vi "Build Metadata String.vi"(11 "Macro Config":T1) -> (3 "Metadata":string)   [LabVIEW 2020, in "MacroAssert.lvlib"]
doc: "Builds a metadata string from <B>Macro Config</B> to be displayed to the user."
uses:
  MacroAssert.lvlib
  CTLs/Macro Config V3.ctl
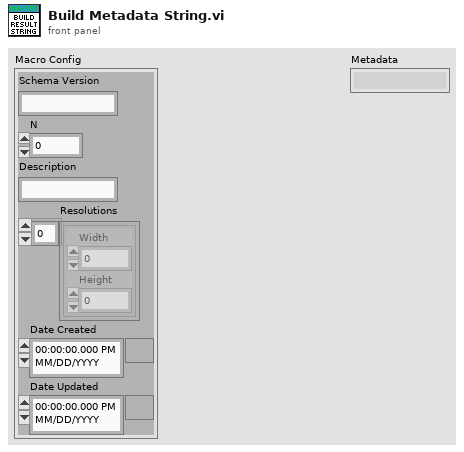
[diagram p1: front panel]
types:
  T1 = typedef "MacroAssert.lvlib/Macro Config V3.ctl" = cluster{"Schema Version":string, "N":i32, "Description":string, "Resolutions":cluster{"Width":i16, "Height":i16}[], "Date Created":timestamp, "Date Updated":timestamp}
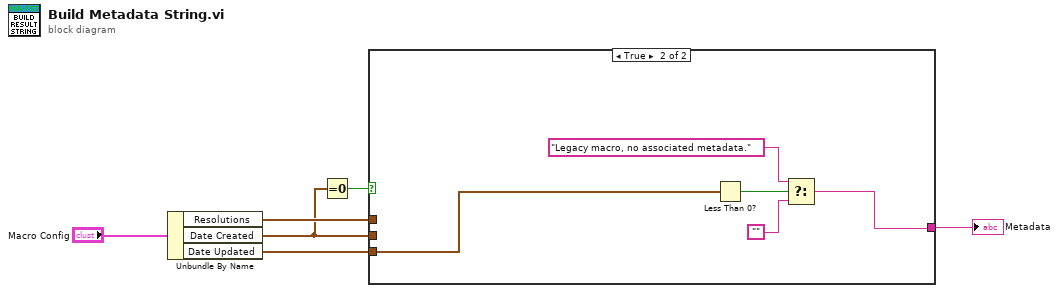
[diagram p0: block diagram]
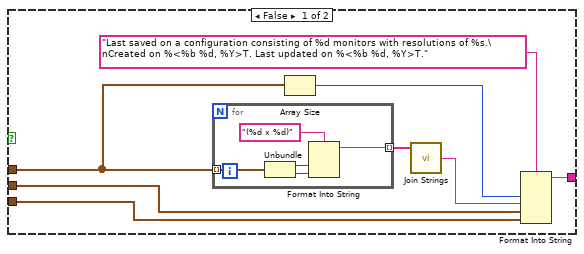
[diagram p2: hidden frame]
diagram:
  n1 = Unbundle By Name("Macro Config") -> ("Resolutions"=w5:cluster{"Width":i16, "Height":i16}[], "Date Created"=w2:timestamp, "Date Updated"=w6:timestamp)
  n2 = Equal To 0?(x=w2) -> (x = 0?=w3:bool)
  n3 = case shown="True" w3 {
    tunnel: w6 -> [w13 w24]
    tunnel: w2 -> [w12 _]
    tunnel: w5 -> [w10 _]
    tunnel: [w7 w20] -> w4
    frame False {
      n4 = for {
        tunnel: w10 -> [w18] mode=indexing
        tunnel: [w15] -> w9 mode=indexing
        n5 = Unbundle(w18) -> ("Width"=w16:i16, "Height"=w17:i16)
        n6 = Format Into String(format string="(%d x %d)", w16, w17) -> (resulting string=w15:string)  [unwired: 2 in, 1 out]
      }
      n7 = Array Size(array=w10) -> (size(s)=w11:i32)
      n8 = call <vilib>:"Join Strings.vi"("Strings In"=w9) -> ("String"=w8:string)  [unwired: 2 in]
      n9 = Format Into String(format string="Last saved on a configuration consisting of %d monitors with resolutions of %s.\nCreated on %<%b %d, %Y>T. Last updated on %<%b %d, %Y>T.", w11, w8, w12, w13) -> (resulting string=w7:string)  [unwired: 2 in, 1 out]
    }
    frame True {
      n10 = Less Than 0?(x=w24) -> (x < 0?=w23:bool)
      n11 = Select(t="Legacy macro, no associated metadata.", s=w23, f="") -> (s? t:f=w20:string)
    }
  }
  "Metadata" <- w4
